vi "relogio.vi"() -> ()   [LabVIEW 2018]
panel:
  in  "Segundos":dbl
  in  "Minutos":dbl
  in  "Horas":dbl
  in  "?":bool
  out "Horas":i32
  out "Minutos":i32
  out "Segundos":i32
  out "Boolean":bool
  in  "stop":bool
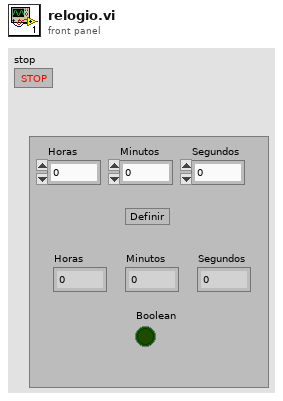
[diagram p1: front panel]
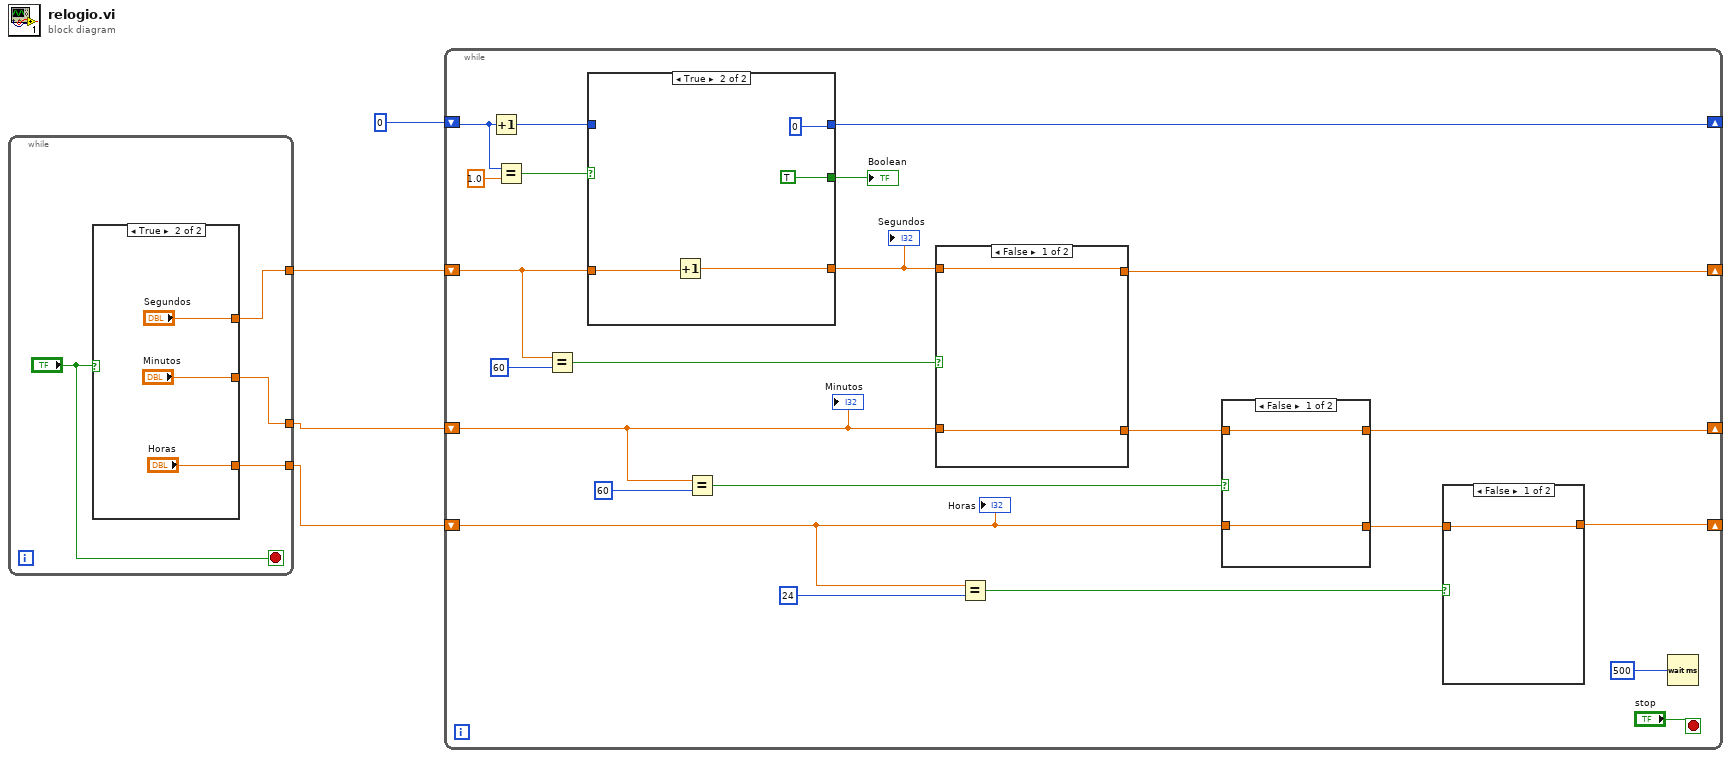
[diagram p0: block diagram]
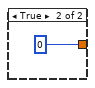
[diagram p3: hidden frame]
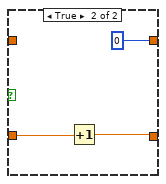
[diagram p4: hidden frame]
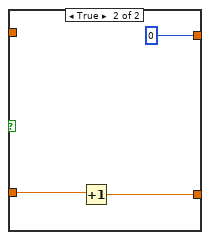
[diagram p5: hidden frame]
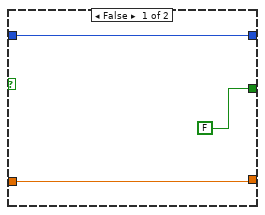
[diagram p6: hidden frame]
diagram:
  n1 = while {
    tunnel: [w8] -> w3
    tunnel: [w7] -> w2
    tunnel: [w6] -> w1
    stop <- "?" stop-if-true
    n2 = case shown="True" "?" {
      tunnel: [_ "Segundos"] -> w8
      tunnel: [_ "Minutos"] -> w7
      tunnel: [_ "Horas"] -> w6
      frame False {
      }
      frame True {
      }
    }
  }
  n3 = while {
    shift-right: [w30] -> _
    shift-left: 0 -> [w33]
    shift-right: [w22] -> _
    shift-left: w3 -> [w26]
    shift-right: [w18] -> _
    shift-left: w2 -> [w21]
    shift-right: [w12] -> _
    shift-left: w1 -> [w16]
    stop <- "stop" stop-if-true
    n4 = Increment(x=w33) -> (x+1=w32:i32)
    n5 = Equal?(x=w33, y=1.0) -> (x = y?=w31:bool)
    n6 = Equal?(x=w26, y=60) -> (x = y?=w24:bool)
    n7 = case shown="True" w31 {
      tunnel: w32 -> [w49 _]
      tunnel: [w49 0] -> w30
      tunnel: [FALSE TRUE] -> w28
      tunnel: w26 -> [w47 w51]
      tunnel: [w47 w50] -> w23
      frame False {
      }
      frame True {
        n8 = Increment(x=w51) -> (x+1=w50:dbl)
      }
    }
    "Boolean" <- w28
    "Segundos" <- w23
    n9 = Equal?(x=w21, y=60) -> (x = y?=w17:bool)
    n10 = case shown="False" w24 {
      tunnel: w23 -> [w43 _]
      tunnel: [w43 0] -> w22
      tunnel: w21 -> [w42 w45]
      tunnel: [w42 w44] -> w19
      frame False {
      }
      frame True {
        n11 = Increment(x=w45) -> (x+1=w44:dbl)
      }
    }
    n12 = Equal?(x=w16, y=24) -> (x = y?=w14:bool)
    n13 = case shown="False" w17 {
      tunnel: w19 -> [w38 _]
      tunnel: [w38 0] -> w18
      tunnel: w16 -> [w37 w40]
      tunnel: [w37 w39] -> w13
      frame False {
      }
      frame True {
        n14 = Increment(x=w40) -> (x+1=w39:dbl)
      }
    }
    n15 = case shown="False" w14 {
      tunnel: w13 -> [w35 _]
      tunnel: [w35 0] -> w12
      frame False {
      }
      frame True {
      }
    }
    n16 = Wait (ms)(milliseconds to wait=u32 500) -> ()  [unwired: 1 out]
    "Minutos" <- w21
    "Horas" <- w16
  }
